vi "Read VISA resource name.vi"(11 "Device in":refnum<class "PIC-Device.lvclass">) -> (2 "VISA resource name":refnum<visa-resource-name>, 3 "Device out":refnum<class "PIC-Device.lvclass">)   [LabVIEW 2020, in "PIC-Device.lvclass"]
uses:
  PIC-Device.lvclass
  PIC-Device.lvclass/PIC-Device.ctl
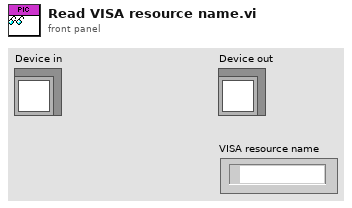
[diagram p1: front panel]
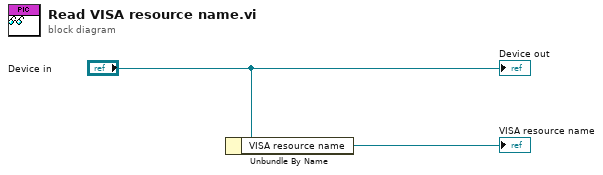
[diagram p0: block diagram]
diagram:
  n1 = Unbundle By Name("Device in") -> ("VISA resource name"=→"VISA resource name":refnum<visa-resource-name>)
  "Device out" <- "Device in"
